vi "Or8Way.vi"(3 "in":bool[](array[boolean])=[FALSE, FALSE, FALSE, FALSE, FALSE, FALSE, FALSE, FALSE, FALSE, FALSE, FALSE, FALSE, FALSE, FALSE, FALSE, FALSE]) -> (1 "out":bool)   [LabVIEW 2014]
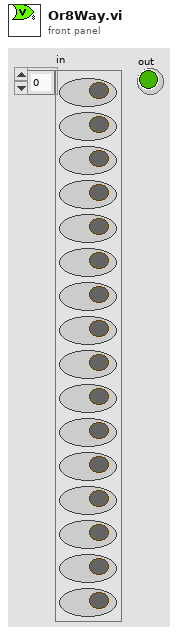
[diagram p1: front panel]
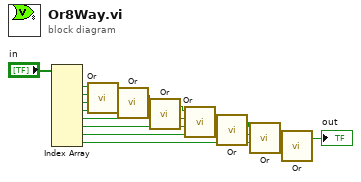
[diagram p0: block diagram]
diagram:
  n1 = Index Array(array="in") -> (element #1=w15:bool, element #2=w14:bool, element #3=w13:bool, element #4=w10:bool, element #5=w9:bool, element #6=w7:bool, element #7=w4:bool, element #8=w2:bool)  [unwired: 8 in]
  n2 = call "Or.vi"("b"=w14, "a"=w15) -> ("out"=w12:bool)  [unwired: 3 in]
  n3 = call "Or.vi"("b"=w13, "a"=w12) -> ("out"=w11:bool)  [unwired: 3 in]
  n4 = call "Or.vi"("b"=w10, "a"=w11) -> ("out"=w8:bool)  [unwired: 3 in]
  n5 = call "Or.vi"("b"=w9, "a"=w8) -> ("out"=w6:bool)  [unwired: 3 in]
  n6 = call "Or.vi"("b"=w7, "a"=w6) -> ("out"=w5:bool)  [unwired: 3 in]
  n7 = call "Or.vi"("b"=w4, "a"=w5) -> ("out"=w3:bool)  [unwired: 3 in]
  n8 = call "Or.vi"("b"=w2, "a"=w3) -> ("out"=→"out":bool)  [unwired: 3 in]
